vi "RSZVB Export User Characterization Data to Touchstone Files.vi"(8 "error in (no error)":errorcluster {"code" format="%.0x"}, 9 "File Name (\"\")":string, 10 "Directory Name (\"\")":string, 11 "VISA session":refnum<visa-resource-name>) -> (0 "error out":errorcluster {"code" format="%.0x"}, 3 "dup VISA session":refnum<visa-resource-name>)   [LabVIEW 2011]
doc: "This VI converts an arbitrary (e.g. user-defined) set of calibration data of the standards in the active calibration\nunit (SYSTem:COMMunicate:RDEVice:AKAL:ADDRess) to Touchstone format and copies it to the specified directory.\n\nRemote-control command(s):\nMMEMory:AKAL:USER:CONVersion '<directory_name>'[,'<file_name>']"
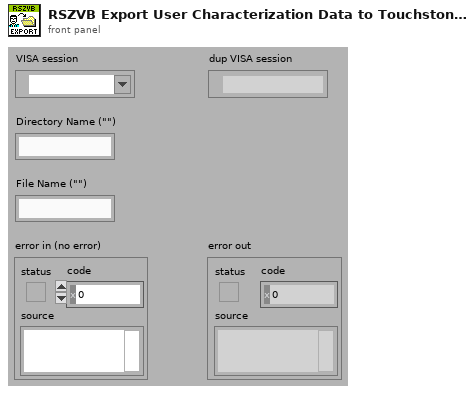
[diagram p1: front panel]
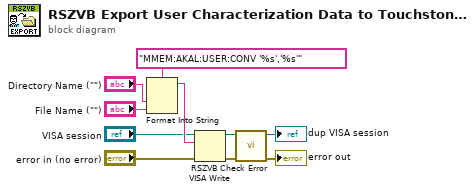
[diagram p0: block diagram]
diagram:
  n1 = Format Into String(format string="MMEM:AKAL:USER:CONV '%s','%s'", "Directory Name (\"\")", "File Name (\"\")") -> (resulting string=w7:string)  [unwired: 2 in, 1 out]
  n2 = VISA Write(VISA resource name="VISA session", write buffer=w7, error in (no error)="error in (no error)") -> (VISA resource name out=w10:refnum<visa-resource-name>, error out=w9:errorcluster)  [unwired: 1 out]
  n3 = call "RSZVB Check Error.vi"("error in (no error)"=w9, "VISA session"=w10) -> ("error out"=→"error out":errorcluster, "dup VISA session"=→"dup VISA session":refnum<visa-resource-name>)  [unwired: 8 in]
